vi "Create Step Parameters.vi"(8 "error in (no error)":errorcluster, 10 "Load current array":dbl[](array[numeric]), 11 "Source voltage array":dbl[][](array[numeric])) -> (0 "error out":errorcluster, 1 "Number of steps":i32, 2 "Load current values":dbl[](array[numeric]), 3 "Source voltage values":dbl[][](array[numeric]))   [LabVIEW 2021, in "Efficiency And Load Regulation with Pin Map.lvlib"]
uses:
  Efficiency And Load Regulation with Pin Map.lvlib
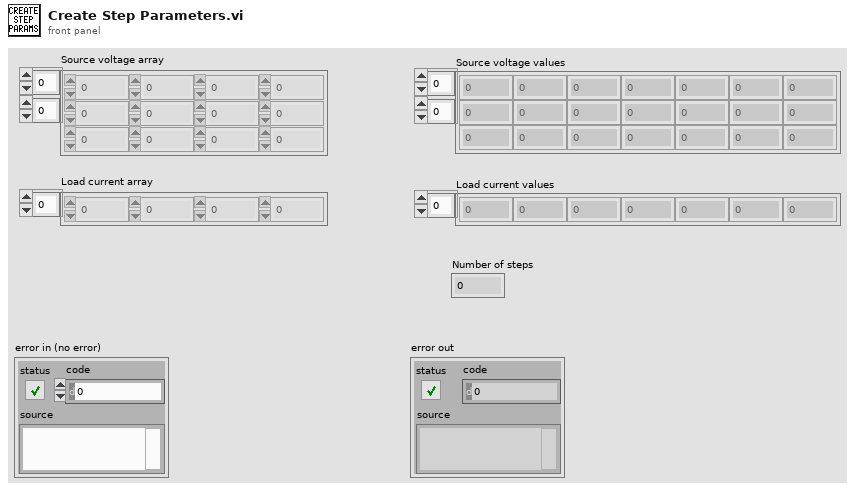
[diagram p1: front panel]
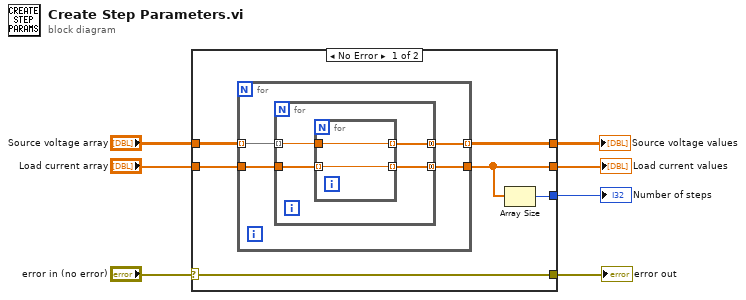
[diagram p0: block diagram]
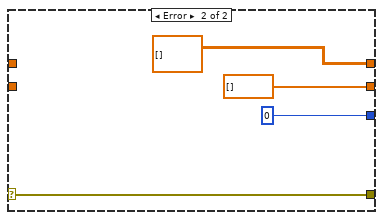
[diagram p2: hidden frame]
diagram:
  n1 = case shown="No Error" "error in (no error)" {
    selector: "error in (no error)" -> [w8 w27]
    tunnel: "Source voltage array" -> [w13 _]
    tunnel: "Load current array" -> [w12 _]
    tunnel: [w11 dbl[][] []] -> w5
    tunnel: [w10 dbl[] []] -> w4
    tunnel: [w9 0] -> w3
    tunnel: [w8 w27] -> w1
    frame No Error {
      n2 = for {
        tunnel: w13 -> [w16] mode=indexing
        tunnel: w12 -> [w17]
        tunnel: [w15] -> w11 mode=indexing
        tunnel: [w14] -> w10
        n3 = for {
          tunnel: w17 -> [w21]
          tunnel: w16 -> [w20] mode=indexing
          tunnel: [w19] -> w15 mode=concatenating
          tunnel: [w18] -> w14 mode=concatenating
          n4 = for {
            tunnel: w21 -> [w22] mode=indexing
            tunnel: w20 -> [w23]
            tunnel: [w23] -> w19 mode=indexing
            tunnel: [w22] -> w18 mode=indexing
          }
        }
      }
      n5 = Array Size(array=w10) -> (size(s)=w9:i32)
    }
    frame Error {
    }
  }
  "Source voltage values" <- w5
  "Load current values" <- w4
  "Number of steps" <- w3
  "error out" <- w1
